vi "Measurement_input_panel.vi"(0 "OK":T4, 2 "setup":T5, 5 "Setup filename":string) -> (11 "Setup filename out":string, 12 "Analysis Info cluster":T8[](array[typedef])=[{"Colour"=0, "Inst type"=enum."Pitot-static tube", "Inst name"="Manometer voltage", "Symbol"="U", "Code name"="", "Extra Info"="U", "Inst Array"=enum."PWA", "Index"=0, "Voltage Index"=0, "Extra Titles"=[], "Extra Values"=[]}, {"Colour"=0, "Inst type"=enum."Pitot-static tube", "Inst name"="Manometer voltage", "Symbol"="U", "Code name"="", "Extra Info"="U", "Inst Array"=enum."PWA", "Index"=0, "Voltage Index"=0, "Extra Titles"=[], "Extra Values"=[]}, {"Colour"=0, "Inst type"=enum."Pitot-static tube", "Inst name"="Manometer voltage", "Symbol"="U", "Code name"="", "Extra Info"="U", "Inst Array"=enum."PWA", "Index"=0, "Voltage Index"=0, "Extra Titles"=[], "Extra Values"=[]}], 19 "Board type":T10=enum."NB-MIO-16H")   [LabVIEW 2010]
uses:
  Controls/Inst_type.ctl
  Controls/Board_Types.ctl
  Controls/Analysis_info_cluster.ctl
  Controls/Instrument_Array.ctl
  Controls/Setup.ctl
  Controls/ok_button.ctl
  Controls/Trigger_Mode.ctl
  Controls/PWA_Data.ctl
  Controls/Post_Process.ctl
  Controls/App_Global.ctl
  Controls/Ch_and_Spans.ctl
  Globals/Meas_global.vi
  Globals/Trav_pos_global.vi
  Globals/Constants_global.vi
  Globals/LDA_meas_global_1.vi
  Globals/Preference_global.vi
panel:
  in  "Select Duplicate Channels":bool
  in  "PWA Data":T1
  out "Inst type":T2
  in  "Edit temp and Press":bool
  out "Abs Press (mbar)":dbl=1013.0 format="%.1f"
  out "Temp (deg C)":dbl=21.0 format="%.1f"
  in  "Trigger mode":T3
  in  "Select Plug Ins":bool
  in  "Sync Delay Time (ms)":dbl=24.0 format="%.2f"
  out "XW Present?":bool
  out "Read Setup File?":bool
  out "Setup File":path
  out "Setup Paths":path[](array[path])
  in  "Select Local ADAM Channels":bool
  out "Local ADAM Channels":string[](array[string])
  in  "stop":bool
  out "Notes":string
  in  "Setup filename selector":u16(ring) items=["Current_Setup.xls", "5168SetupTakeZeroes.xls", "5168FIDRawVoltsSanityCheck.xls", "5168Setup6min.xls", "5168Setup5min.xls", "5168Setup4min.xls", "5168Setup3min.xls", "5168SetupTapped1to1cal.xls", "5168SetupTappedNoPuffs1to1cal.xls", "5168SetupTappedNoPuffs.xls", "5168SetupTapped.xls", "5168Setup2.xls", "5168FIDcheck.xls", "5168Setup1.xls"]
  in  "Synchronise Analogue channels with LDA":bool
  in  "LDA set up":T6={"dimensions"=enum."2D", "Arrival spacing"=FALSE, "Transit time"=FALSE}
  in  "LDA data":enum16{"No LDA data", "Take LDA data"}(ring)=enum."Take LDA data"
  in  "Cross wire":T7(ring)
  in  "Acquisition Method":T10=enum."NB-MIO-16H"
  in  "No of Analogue inst":i32=1
  in  "Ch & spans choices":T11(array[cluster]) {"D" format="%.2f"; "Ch No" min=0; "low limit" min=-10 max=10 format="%.2f"; "high limit" min=-10 max=10 format="%.2f"}
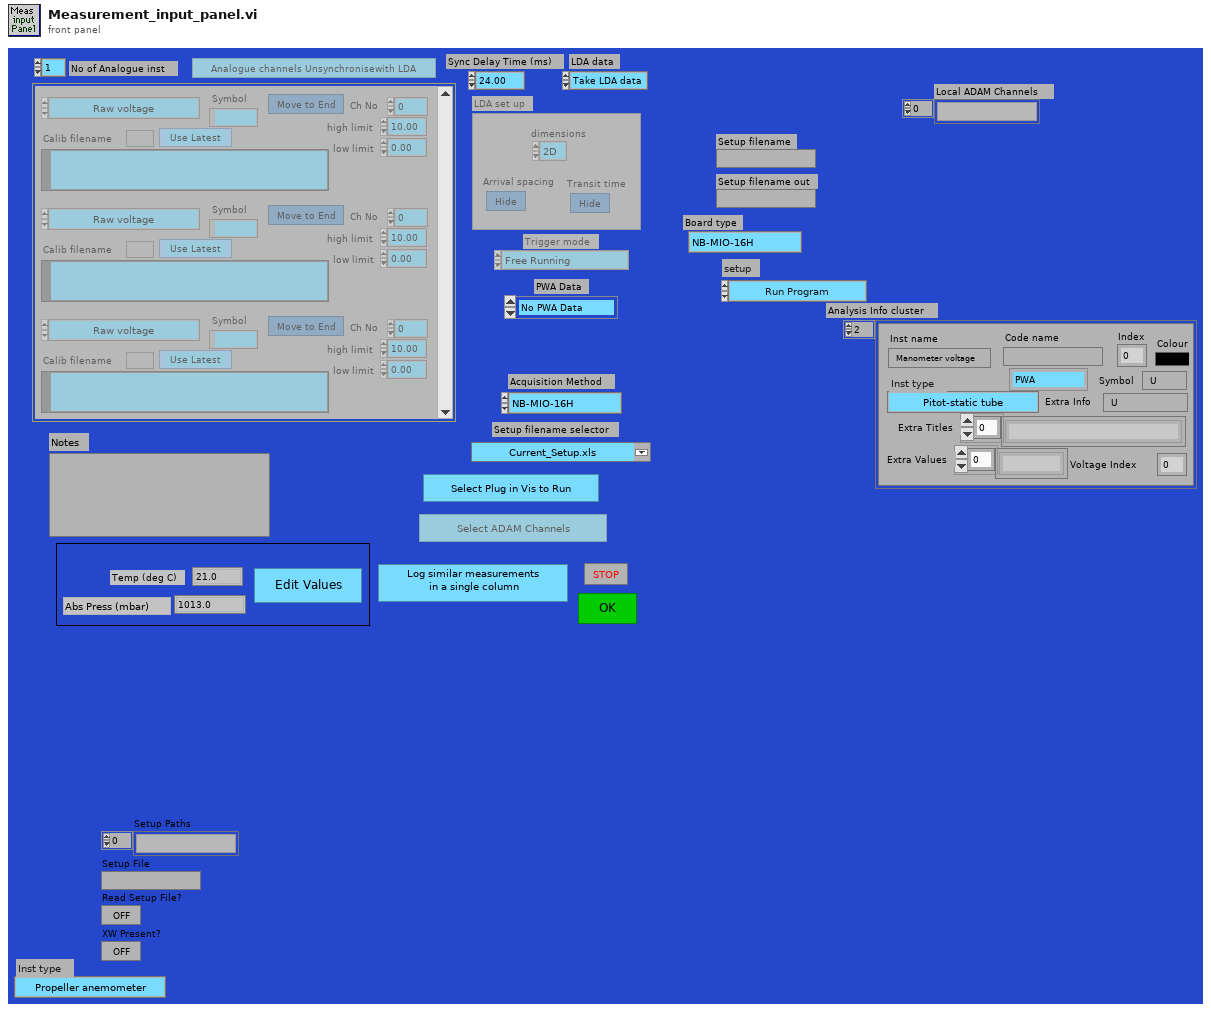
[diagram p1: front panel]
types:
  T1 = typedef "PWA_Data.ctl" = enum16{"No PWA Data", "One Ch PWA"}
  T2 = typedef "Inst_type.ctl" = enum16{"Propeller anemometer", "Raw voltage", "Pressure Transducer", "Pitot-static tube", "Preston tube", "Hot wire", "Cross wire 1", "Cross wire 2", "Generic Linear", "Generic Polynomial", "Generic BackPoly", "Fast FID", "Thermocouple", "Cold wire", "Pulsed Wire", "LDA Vel", "LDA Tran time", "LDA Arr time"}
  T3 = typedef "Trigger_Mode.ctl" = enum16{"Free Running", "Start on Trigger", "Trigger Every Block", "Trigger Every Sample"}
  T4 = typedef "ok_button.ctl" = bool
  T5 = typedef "Setup.ctl" = enum16{"Run Program", "Show Setup", "Save Current Setup", "Setup Front Panel"}
  T6 = cluster{"dimensions":enum16{"1D", "2D"}, "Arrival spacing":bool, "Transit time":bool}
  T7 = enum16{"2nd component as calculated", "2nd component multipled by -1"}
  T8 = typedef "Analysis_info_cluster.ctl" = cluster{"Colour":u32, "Inst type":T2, "Inst name":string, "Symbol":string, "Code name":string, "Extra Info":string, "Inst Array":T9, "Index":i32, "Voltage Index":i32, "Extra Titles":string[], "Extra Values":string[]}
  T9 = typedef "Instrument_Array.ctl" = enum16{"PWA", "LDA", "Analogue"}
  T10 = typedef "Board_Types.ctl" = enum16{"Simulate", "NB-MIO-16H", "PCI-MIO-16E", "6000E Series", "USB-92xx", "ADC488", "Lab-NB", "NB-DIO-24", "NI-DAQmx", "Local ADAM", "Server Channels"}
  T11 = cluster{"high limit":sgl, "low limit":sgl, "Ch No":i16, "Calib filename":path, "Inst type":T2, "Symbol":string, "Move channel":bool, "Use Latest":bool, "D":dbl, "Ch Name":string}[]
  T12 = typedef "Post_Process.ctl" = enum16{"Take New Data", "Post Process Raw Data File"}
  T13 = cluster{"high limit (10V)":sgl, "low limit (-10V)":sgl, "Ch No":i16, "Calib filename":path, "Inst type":T2, "Symbol":string, "Move channel":bool, "Use Latest":bool, "D":dbl, "Ch Name":string}
  T14 = typedef "App_Global.ctl" = enum16{"Read Global", "Write to Global", "Initialise Array"}
  T15 = typedef "Ch_and_Spans.ctl" = cluster{"high limit (10V)":sgl, "low limit (-10V)":sgl, "Ch No":i16, "Var name":string, "Use Latest Calib":bool}
  T16 = enum16{"Zero or one", "One", "Zero or more", "One or more"}
  T17 = typedef "Traverse_cluster.ctl" = cluster{"Start X":dbl, "Start Y":dbl, "Start Z":dbl, "End X":dbl, "End Y":dbl, "End Z":dbl, "No. of pts.":i32, "Spacing":T18, "Filename":path, "Tunnel Speed":dbl, "Averaging time (min)":dbl, "Extra Commands":string, "Specific Arguments":string, "Emission Rate (l/min)":dbl, "Trace Gas Concentration (%)":dbl, "Density Ratio":string, "Comments":string, "Row No":i32, "Row Type Selector":T19, "Completion time":string, "Row Duration (mins)":dbl, "No. of Valid pts.":i32, "Meas Setup File":string}
  T18 = typedef "Spacing.ctl" = enum16{"Linear", "Log", "Gauss", "Specified", "N/A"}
  T19 = typedef "Multi_run_mode.ctl" = enum16{"Move Traverse Only", "Set Tunnel Speed Only", "Set Source Only", "Set Measurement Conditions", "Single Measurement", "Vertical Profile", "Lateral Profile", "Longitudinal Profile", "Explore Volume", "Multi-Axis Profile", "Auto Calibrate", "Meas Fast FID Bkgnd", "Check Beam Power", "Scanning Valve Measurement", "Run VI Named:", "Set ADAM Ch", "Wait (minutes)", "Send Message", "Synchronize With:", "Fall Back to this Row", "Turn Off Row Repeating", "Blank Row"}
  T20 = cluster{"high limit (10V)":sgl, "low limit (-10V)":sgl, "Ch No":i16, "Calib filename":path, "Inst type":T2, "Symbol":string, "Move channel":bool, "Use Latest":bool, "D":dbl, "Ch Name":string}[]
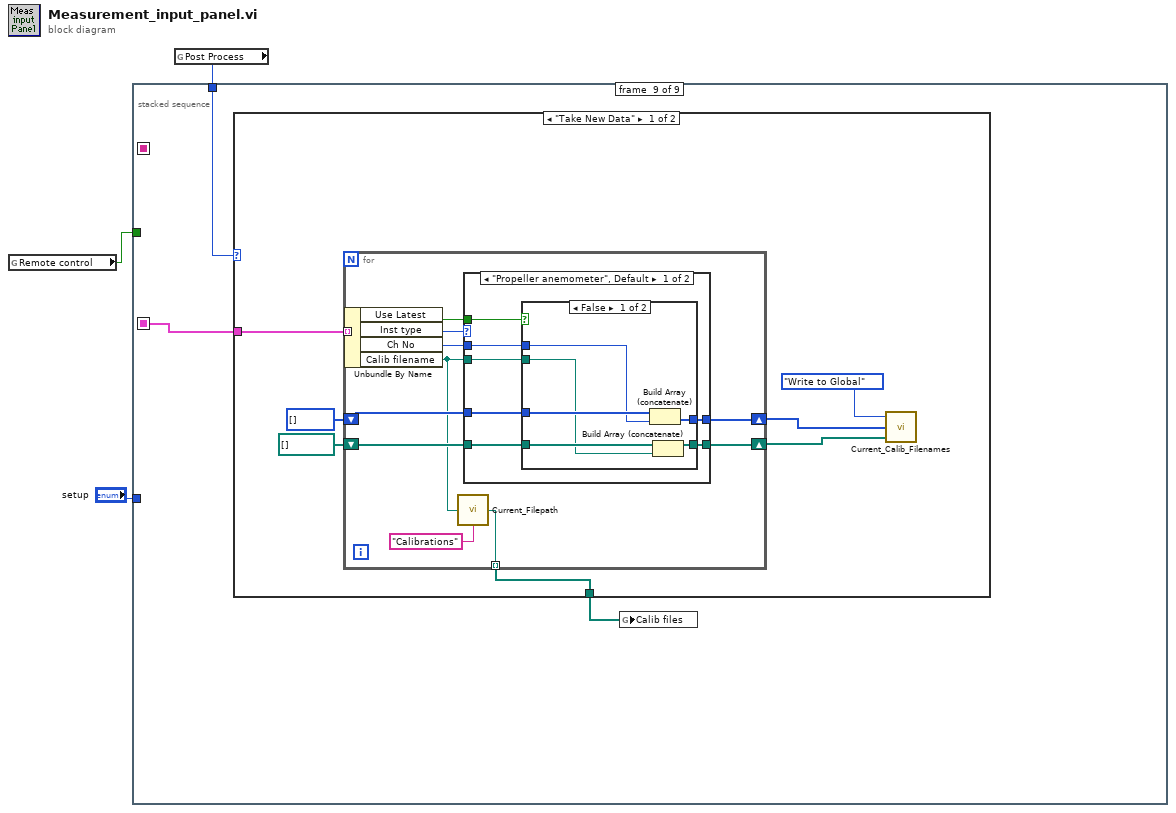
[diagram p0: block diagram]
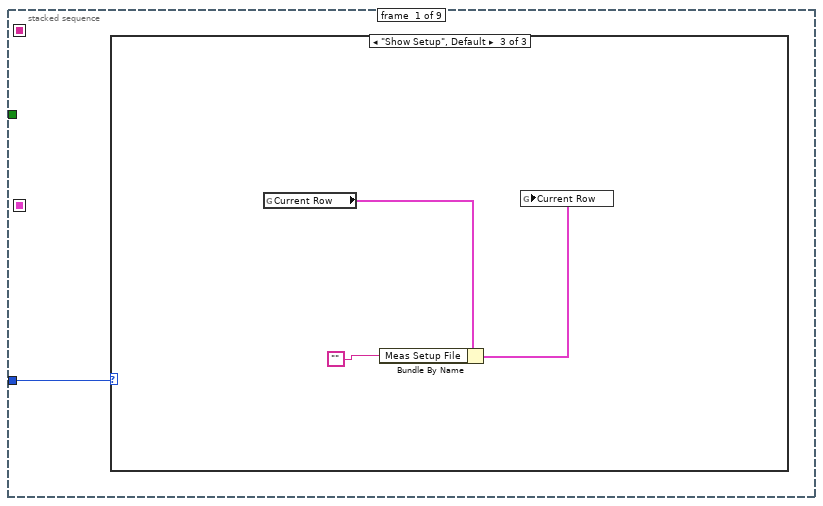
[diagram p2: hidden frame]
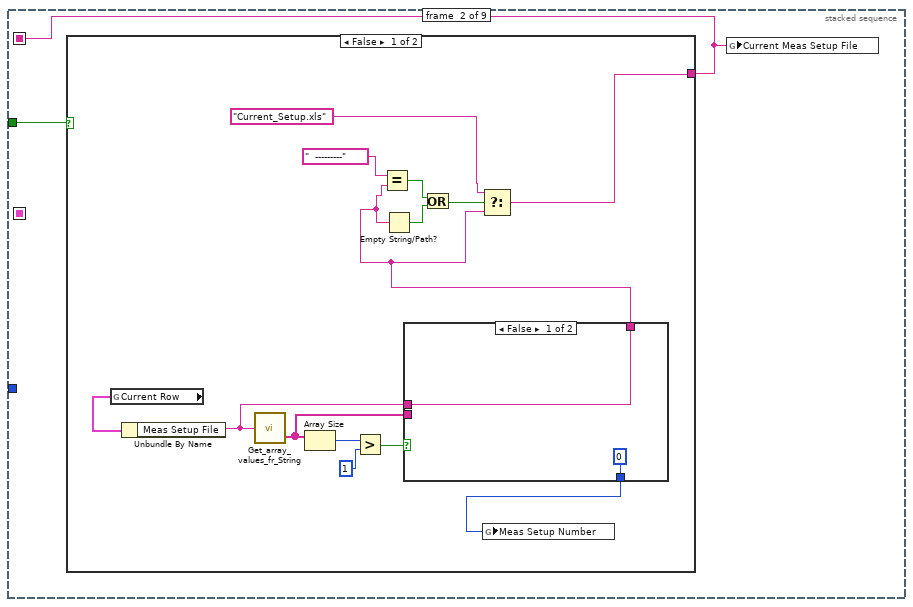
[diagram p5: hidden frame]
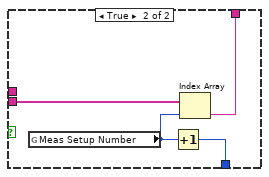
[diagram p6: hidden frame]
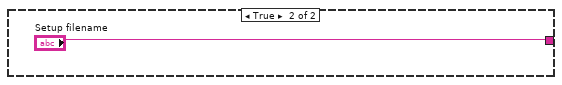
[diagram p7: hidden frame]
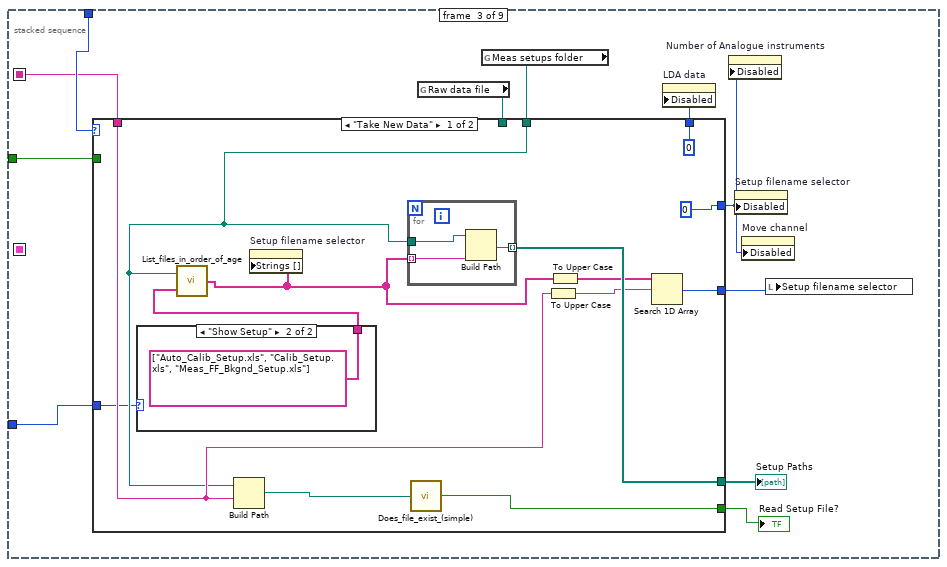
[diagram p8: hidden frame]
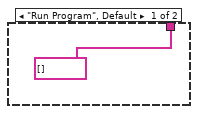
[diagram p9: hidden frame]
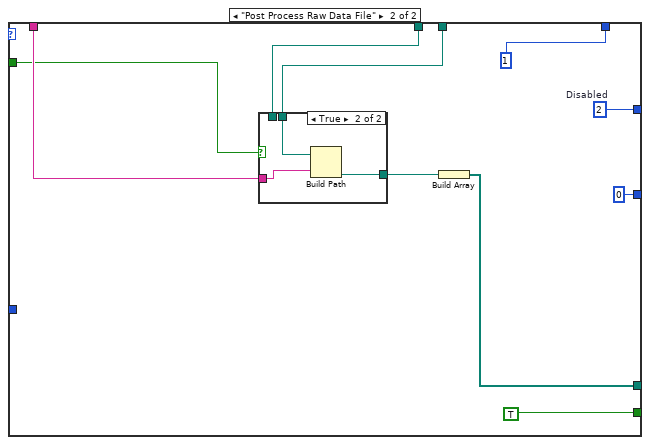
[diagram p10: hidden frame]
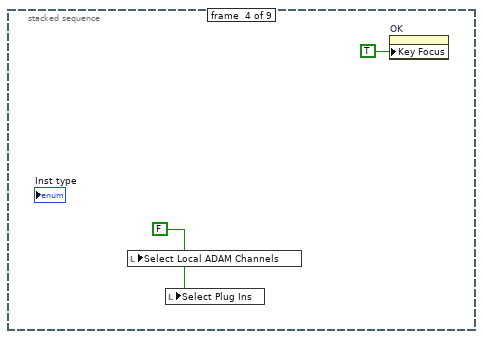
[diagram p12: hidden frame]
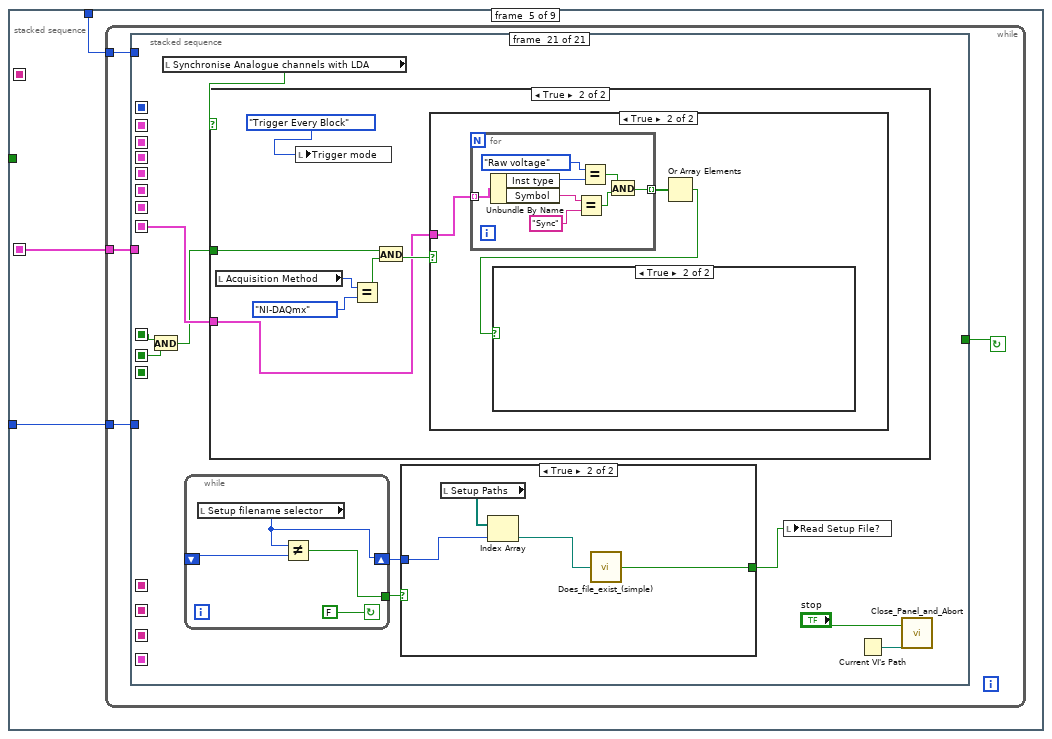
[diagram p13: hidden frame]
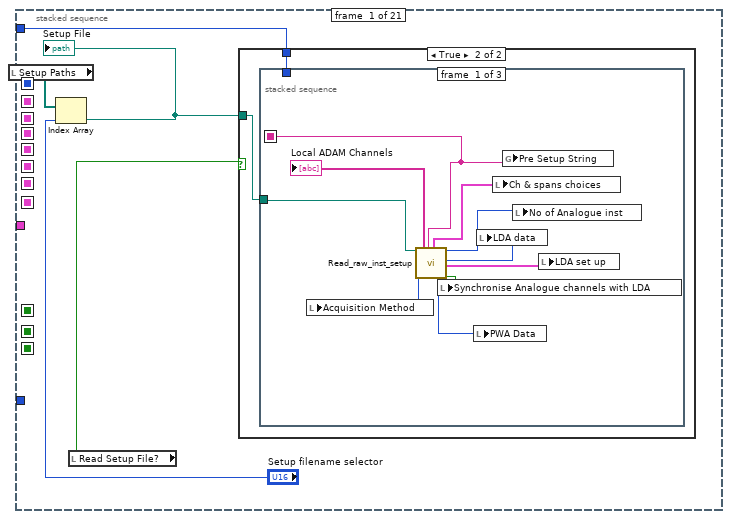
[diagram p14: hidden frame]
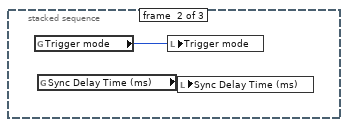
[diagram p16: hidden frame]
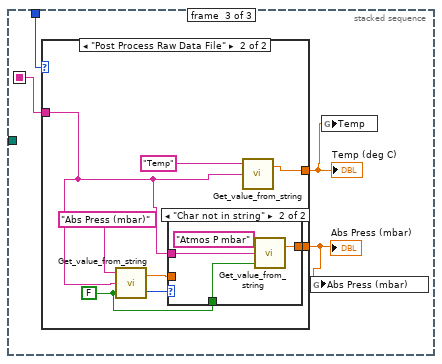
[diagram p17: hidden frame]
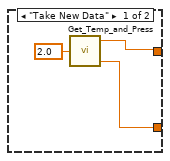
[diagram p18: hidden frame]
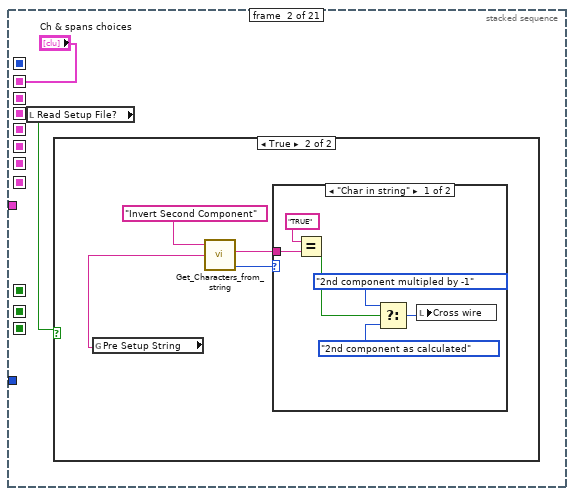
[diagram p20: hidden frame]
diagram:
  n1 = global read "Meas_global.vi" "Remote control"() -> (w1:bool)
  n2 = global read "Meas_global.vi" "Post Process"() -> (w3:T12)
  n3 = stacked-sequence {
    seq-local: [_ _ _ _ w78 _ _ _ _] -> [_ _ _ _ _ _ w762 _ w888]
    seq-local: [_ w8 _ _ _ _ _ _ _] -> [_ _ w31 _ _ _ w761 _ _]
    tunnel: w3 -> [_ _ w41 _ w77 _ _ _ w887]
    tunnel: "setup" -> [w4 _ w33 _ w76 _ w763 _ _]
    tunnel: w1 -> [_ w9 w32 _ _ _ _ _ _]
    frame #0 {
      n4 = case shown="\"Show Setup\", Default" w4 {
        frame "Run Program" {
        }
        frame "Setup Front Panel" {
        }
        frame "Show Setup", Default {
          n5 = global read "Trav_pos_global.vi" "Current Row"() -> (w7:T17)
          n6 = Bundle By Name(cluster=w7, "Meas Setup File"="") -> (w6:T17)
          n7 = global write "Trav_pos_global.vi" "Current Row"(w6) -> ()
        }
      }
    }
    frame #1 {
      n8 = case shown="False" w9 {
        tunnel: [w22 "Setup filename"] -> w8
        frame False {
          n9 = global read "Trav_pos_global.vi" "Current Row"() -> (w18:T17)
          n10 = Unbundle By Name(w18) -> ("Meas Setup File"=w12:string)
          n11 = call "Get_array_values_fr_String.vi"("String Value"=w12) -> ("String array"=w11:string[])  [unwired: 1 out]
          n12 = Array Size(array=w11) -> (size(s)=w16:i32)
          n13 = Greater?(x=w16, y=1) -> (0:w14:bool)
          n14 = case shown="False" w14 {
            tunnel: [w25 w28] -> w13
            tunnel: w12 -> [w25 _]
            tunnel: w11 -> [_ w29]
            tunnel: [0 w26] -> w10
            frame False {
            }
            frame True {
              n15 = global read "Trav_pos_global.vi" "Meas Setup Number"() -> (w27:i32)
              n16 = Increment(x=w27) -> (x+1=w26:i32)
              n17 = Index Array(array=w29, index=w27) -> (element=w28:string)
            }
          }
          n18 = Equal?(x="  ---------" ("f"), y=w13) -> (x = y?=w21:bool)
          n19 = Empty String/Path?(string/path=w13) -> (empty?=w20:bool)
          n20 = Or(x=w21, y=w20) -> (x .or. y?=w17:bool)
          n21 = Select(t="Current_Setup.xls", s=w17, f=w13) -> (s? t:f=w22:string)
          n22 = global write "Trav_pos_global.vi" "Meas Setup Number"(w10) -> ()
        }
        frame True {
        }
      }
      n23 = global write "Trav_pos_global.vi" "Current Meas Setup File"(w8) -> ()
    }
    frame #2 {
      n24 = global read "Meas_global.vi" "Raw data file"() -> (w38:path)
      n25 = global read "Constants_global.vi" "Meas setups folder"() -> (w36:path)
      n26 = case shown="\"Take New Data\"" w41 {
        tunnel: [w52 w65] -> w35
        tunnel: [w46 TRUE ("exists")] -> w34
        tunnel: [u8 0 ("Disabled") w61] -> w37
        tunnel: [u8 0 ("Disabled") u8 1 ("Disabled")] -> w40
        tunnel: w31 -> [w51 w67]
        tunnel: [w53 0 ("index of element")] -> w39
        tunnel: w36 -> [w48 w68]
        tunnel: w38 -> [_ w63]
        tunnel: w33 -> [w42 _]
        tunnel: w32 -> [_ w60]
        frame "Take New Data" {
          n27 = case shown="\"Show Setup\"" w42 {
            tunnel: [string[] [] ("file names") string[] ["Auto_Calib_Setup.xls", "Calib_Setup.xls", "Meas_FF_Bkgnd_Setup.xls"] ("file names")] -> w44
            frame "Run Program", Default {
            }
            frame "Show Setup" {
            }
          }
          n28 = call "List_files_in_order_of_age.vi"("Files to Hide"=w44, "Folder"=w48) -> ("file names"=w43:string[])
          n29 = Build Path(base path=w48, name or relative path=w51) -> (appended path=w47:path)
          n30 = property on="Setup filename selector" class="Ring (strict)"("Strings []"=w43) -> ()  [unwired: 2 in, 2 out]
          n31 = for {
            tunnel: [w57] -> w52 mode=indexing
            tunnel: w48 -> [w58]
            tunnel: w43 -> [w59] mode=indexing
            n32 = Build Path(base path=w58, name or relative path=w59) -> (appended path=w57:path)
          }
          n33 = call "Does_file_exist_(simple).vi"("Pathname"=w47) -> ("exists?"=w46:bool)
          n34 = To Upper Case(1:w51) -> (0:w49:string)
          n35 = To Upper Case(1:w43) -> (0:w50:string[])
          n36 = Search 1D Array(1D array=w50, element=w49) -> (index of element=w53:i32)  [unwired: 1 out]
        }
        frame "Post Process Raw Data File" {
          w61 = u8 2  # Disabled
          n37 = case shown="True" w60 {
            tunnel: w68 -> [_ w73]
            tunnel: w67 -> [_ w72]
            tunnel: [w70 w71] -> w66
            tunnel: w63 -> [w70 _]
            frame False {
            }
            frame True {
              n38 = Build Path(base path=w73, name or relative path=w72) -> (appended path=w71:path)
            }
          }
          n39 = Build Array(w66) -> (w65:path[])
        }
      }
      "Setup Paths" <- w35
      "Read Setup File?" <- w34
      n40 = property on="LDA data" class="Enum (strict)"("Disabled"=w40) -> ()  [unwired: 2 in, 2 out]
      n41 = property on="Number of Analogue instruments" class="DigNum (strict)"("Disabled"=w37) -> ()  [unwired: 2 in, 2 out]
      n42 = property on="Setup filename selector" class="Ring (strict)"("Disabled"=w37) -> ()  [unwired: 2 in, 2 out]
      n43 = property on="Move channel" class="Bool (strict)"("Disabled"=w37) -> ()  [unwired: 2 in, 2 out]
      n44 = local write "Setup filename selector"(w39) -> ()
    }
    frame #3 {
      w75 = FALSE ("Select Local ADAM Channels")
      n45 = local write "Select Local ADAM Channels"(w75) -> ()
      n46 = local write "Select Plug Ins"(w75) -> ()
      n47 = property on="OK" class="Bool"("Key Focus"=TRUE) -> ()  [unwired: 2 in, 2 out]
    }
    frame #4 {
      n48 = while {
        tunnel: w76 -> [w79]
        tunnel: w77 -> [w80]
        tunnel: [w82] -> w78
        stop <- w81 continue-if-true
        n49 = stacked-sequence {
          seq-local: [_ _ _ _ _ _ _ _ w270 _ _ _ _ _ _ _ _ _ _ _ _] -> [_ _ _ _ _ _ _ _ _ w337 _ _ _ _ _ _ _ _ _ _ _]
          seq-local: [_ _ _ w159 _ _ _ _ _ _ _ _ _ _ _ _ _ _ _ _ _] -> [_ _ _ _ _ w212 w247 w266 w271 _ _ _ _ _ _ _ _ _ _ _ _]
          seq-local: [_ _ _ _ _ w217 _ _ _ _ _ _ _ _ _ _ _ _ _ _ _] -> [_ _ _ _ _ _ _ _ w272 _ _ _ _ _ _ _ _ _ _ _ _]
          seq-local: [_ _ _ _ _ _ _ _ _ w336 _ _ _ _ _ _ _ _ _ _ _] -> [_ _ _ _ _ _ _ _ _ _ w370 w418 w461 _ _ _ _ _ _ _ _]
          seq-local: [_ _ _ _ _ _ _ _ _ _ w368 _ _ _ _ _ _ _ _ _ _] -> [_ _ _ _ _ _ _ _ _ _ _ w413 _ _ _ _ _ _ _ _ w721]
          seq-local: [_ _ _ _ _ _ _ _ _ _ _ _ _ w490 _ _ _ _ _ _ _] -> [_ _ _ _ _ _ _ _ _ _ _ _ _ _ w509 _ _ _ _ _ _]
          seq-local: [_ _ _ _ _ _ _ _ _ _ _ _ _ _ w505 _ _ _ _ _ _] -> [_ _ _ _ _ _ _ _ _ _ _ _ _ _ _ w531 w537 w600 _ w697 w722]
          seq-local: [_ _ _ _ _ _ _ _ _ _ _ w417 _ _ _ _ _ _ _ _ _] -> [_ _ _ _ _ _ _ _ _ _ _ _ _ w487 _ _ _ _ _ _ _]
          seq-local: [_ _ _ _ _ _ _ _ _ _ _ _ w460 _ _ _ _ _ _ _ _] -> [_ _ _ _ _ _ _ _ _ _ _ _ _ w486 _ _ _ _ _ _ _]
          seq-local: [_ _ _ _ _ _ _ _ _ w330 _ _ _ _ _ _ _ _ _ _ _] -> [_ _ _ _ _ _ _ _ _ _ w367 w414 _ _ _ _ _ _ _ _ w720]
          seq-local: [_ _ _ _ _ _ _ _ _ _ _ _ _ _ _ _ w536 _ _ _ _] -> [_ _ _ _ _ _ _ _ _ _ _ _ _ _ _ _ _ w603 _ _ _]
          seq-local: [_ _ _ _ _ _ _ _ _ _ _ _ _ _ _ _ w535 _ _ _ _] -> [_ _ _ _ _ _ _ _ _ _ _ _ _ _ _ _ _ w602 _ _ _]
          seq-local: [_ _ _ _ _ _ _ _ _ _ _ _ _ _ _ _ w534 _ _ _ _] -> [_ _ _ _ _ _ _ _ _ _ _ _ _ _ _ _ _ w601 _ _ _]
          seq-local: [_ _ _ _ _ _ _ _ _ _ _ _ _ _ _ _ _ w599 _ _ _] -> [_ _ _ _ _ _ _ _ _ _ _ _ _ _ _ _ _ _ w641 _ _]
          seq-local: [_ "Ch & spans choices" _ _ _ _ _ _ _ _ _ _ _ _ _ _ _ _ _ _ _] -> [_ _ _ w142 _ _ _ _ _ _ _ _ _ _ _ w530 _ _ _ _ _]
          tunnel: [_ _ _ _ _ _ _ _ _ _ _ _ _ _ w505 _ _ _ _ _ _] -> w82
          tunnel: [_ _ _ _ _ _ _ _ _ _ _ w415 _ _ _ _ _ _ _ _ _] -> w81
          tunnel: w80 -> [w83 _ w134 w154 _ _ _ _ _ w331 _ w412 _ w489 _ _ _ _ _ w698 _]
          tunnel: w79 -> [_ _ _ _ w198 _ _ _ _ _ _ _ _ w488 _ _ _ _ w643 _ _]
          frame #0 {
            n50 = local read "Setup Paths"() -> (w86:path[])
            n51 = Index Array(array=w86, index="Setup filename selector") -> (element=w87:path)
            "Setup File" <- w87
            n52 = local read "Read Setup File?"() -> (w85:bool)
            n53 = case shown="True" w85 {
              tunnel: w87 -> [_ w89]
              tunnel: w83 -> [_ w88]
              frame False {
              }
              frame True {
                n54 = stacked-sequence {
                  seq-local: [w92 _ _] -> [_ _ w104]
                  tunnel: w89 -> [w95 _ _]
                  tunnel: w88 -> [_ _ w105]
                  frame #0 {
                    n55 = call "Read_raw_inst_setup.vi"("Setup file"=w95) -> ("Board type"=w97:T10, "Local ADAM Channels"=→"Local ADAM Channels":string[], "Setup string"=w92:string, "Ch & spans choices"=w91:T20, "PWA Data"=w90:T1, "Number of Analogue instruments"=w99:i32, "LDA data"=w98:enum16{"No LDA data", "Take LDA data"}, "LDA set up"=w94:T6, "Synchronise Analogue channels with LDA"=w96:bool)  [unwired: 10 out]
                    n56 = local write "Acquisition Method"(w97) -> ()
                    n57 = local write "Synchronise Analogue channels with LDA"(w96) -> ()
                    n58 = local write "PWA Data"(w90) -> ()
                    n59 = local write "LDA data"(w98) -> ()
                    n60 = local write "Ch & spans choices"(w91) -> ()
                    n61 = global write "Meas_global.vi" "Pre Setup String"(w92) -> ()
                    n62 = local write "No of Analogue inst"(w99) -> ()
                    n63 = local write "LDA set up"(w94) -> ()
                  }
                  frame #1 {
                    n64 = global read "Meas_global.vi" "Trigger mode"() -> (w100:T3)
                    n65 = global read "LDA_meas_global_1.vi" "Sync Delay Time (ms)"() -> (w101:dbl)
                    n66 = local write "Trigger mode"(w100) -> ()
                    n67 = local write "Sync Delay Time (ms)"(w101) -> ()
                  }
                  frame #2 {
                    n68 = case shown="\"Post Process Raw Data File\"" w105 {
                      tunnel: w104 -> [_ w111]
                      tunnel: [w106 w110] -> w102
                      tunnel: [w107 w109] -> w103
                      frame "Take New Data" {
                        n69 = call "Get_Temp_and_Press.vi"("Averaging time (mins)"=2.0) -> ("Abs Press (mbar)"=w106:dbl, "Temperature"=w107:dbl)  [unwired: 3 out]
                      }
                      frame "Post Process Raw Data File" {
                        w113 = FALSE ("Show Dialog?")
                        n70 = call "Get_value_from_string.vi"("Show Dialog?"=w113, "Input string"=w111, "Variable name"="Abs Press (mbar)") -> ("Status"=w115:enum16{"Char in string", "Char not in string"}, "Value"=w114:dbl)
                        n71 = case shown="\"Char not in string\"" w115 {
                          tunnel: [w117 w120] -> w110
                          tunnel: w114 -> [w117 _]
                          tunnel: w113 -> [_ w119]
                          tunnel: w111 -> [_ w118]
                          frame "Char in string" {
                          }
                          frame "Char not in string" {
                            n72 = call "Get_value_from_string.vi"("Show Dialog?"=w119, "Input string"=w118, "Variable name"="Atmos P mbar") -> ("Value"=w120:dbl)  [unwired: 1 out]
                          }
                        }
                        n73 = call "Get_value_from_string.vi"("Input string"=w111, "Variable name"="Temp") -> ("Value"=w109:dbl)  [unwired: 1 in, 1 out]
                      }
                    }
                    "Abs Press (mbar)" <- w102
                    "Temp (deg C)" <- w103
                    n74 = global write "Meas_global.vi" "Abs Press (mbar)"(w102) -> ()
                    n75 = global write "Meas_global.vi" "Temp"(w103) -> ()
                  }
                }
              }
            }
          }
          frame #1 {
            n76 = local read "Read Setup File?"() -> (w123:bool)
            n77 = case shown="True" w123 {
              frame False {
              }
              frame True {
                n78 = global read "Meas_global.vi" "Pre Setup String"() -> (w126:string)
                n79 = call "Get_Characters_from_string.vi"("Input string"=w126, "Variable name"="Invert Second Component") -> ("Status"=w125:enum16{"Char in string", "Char not in string"}, "Value"=w124:string)  [unwired: 1 in]
                n80 = case shown="\"Char in string\"" w125 {
                  tunnel: w124 -> [w133 _]
                  frame "Char in string" {
                    n81 = Equal?(x="TRUE", y=w133) -> (x = y?=w129:bool)
                    n82 = Select(t=T7."2nd component multipled by -1" ("Cross wire/LDA"), s=w129, f=T7."2nd component as calculated" ("Cross wire/LDA")) -> (s? t:f=w131:T7)
                    n83 = local write "Cross wire"(w131) -> ()
                  }
                  frame "Char not in string" {
                  }
                }
              }
            }
          }
          frame #2 {
            n84 = case shown="True" "Edit temp and Press" {
              tunnel: w134 -> [_ w136]
              frame False {
              }
              frame True {
                n85 = case shown="\"Take New Data\"" w136 {
                  frame "Take New Data" {
                    n86 = stacked-sequence {
                      frame #0 {
                        w137 = TRUE  # Wait until done
                        n87 = call "Run_Enter_Temp.vi"("Wait until done"=w137) -> ()  [unwired: 1 out]
                      }
                      frame #1 {
                        n88 = call "Get_Temp_and_Press.vi"("Averaging time (mins)"=2.0) -> ("Abs Press (mbar)"=w138:dbl, "Temperature"=w139:dbl)  [unwired: 3 out]
                        n89 = local write "Temp (deg C)"(w139) -> ()
                        n90 = local write "Abs Press (mbar)"(w138) -> ()
                      }
                    }
                  }
                  frame "Post Process Raw Data File" {
                  }
                }
              }
            }
          }
          frame #3 {
            w150 = u8 0  # Disabled
            n91 = local read "Read Setup File?"() -> (w141:bool)
            n92 = Equal?(x=w154, y=Post_Process."Take New Data" ("Post Process")) -> (x = y?=w153:bool)
            n93 = local read "Acquisition Method"() -> (w147:T10)
            n94 = Equal?(x=w147, y=Board_Types."Local ADAM" ("Board type")) -> (x = y?=w144:bool)
            n95 = Equal?(x=Board_Types."Server Channels" ("Board type"), y=w147) -> (x = y?=w145:bool)
            n96 = Or(x=w144, y=w145) -> (x .or. y?=w143:bool)
            n97 = And(x=w141, y=w143) -> (x .and. y?=w158:bool)
            n98 = Or(x="Select Local ADAM Channels", y=w158) -> (x .or. y?=w151:bool)
            n99 = And(x=w153, y=w151) -> (x .and. y?=w152:bool)
            n100 = case shown="True" w152 {
              tunnel: [w161 w164] -> w159
              tunnel: w142 -> [w161 w165]
              tunnel: "Select Local ADAM Channels" -> [_ w163]
              tunnel: w144 -> [_ w162]
              frame False {
              }
              frame True {
                n101 = local read "Local ADAM Channels"() -> (w167:string[])
                n102 = stacked-sequence {
                  seq-local: [_ w176 _ _ _] -> [_ _ w182 w195 _]
                  seq-local: [_ w180 _ _ _] -> [_ _ w186 _ _]
                  seq-local: [T13 {"high limit (10V)"=10.0, "low limit (-10V)"=0.0, "Ch No"=0, "Calib filename"=path "", "Inst type"=enum."Raw voltage", "Symbol"="", "Move channel"=FALSE, "Use Latest"=FALSE, "D"=0.0, "Ch Name"=""} _ _ _ _] -> [_ w172 _ _ _]
                  seq-local: [_ w169 _ _ _] -> [_ _ w184 _ _]
                  tunnel: w167 -> [_ w179 _ _ _]
                  tunnel: [_ w180 _ _ _] -> w166
                  tunnel: w165 -> [_ w171 _ _ _]
                  tunnel: [_ _ w185 _ _] -> w164
                  tunnel: w163 -> [_ w181 _ _ w196]
                  tunnel: w162 -> [_ w177 w183 _ _]
                  frame #0 {
                  }
                  frame #1 {
                    n103 = Array Size(array=w171) -> (size(s)=w174:i32)
                    n104 = Array Subset(array=w179, length=w174) -> (w178:string[])  [unwired: 1 in]
                    n105 = call "Get_local_ADAM_Chs.vi"("Local ADAM?"=w177, "Show setup"=w181, "Desired Local ADAM Channels"=w178) -> ("Choosen Channels"=w180:string[], "Ch Indicies Choosen"=w176:i32[])
                    n106 = Array Size(array=w176) -> (size(s)=w175:i32)
                    n107 = Subtract(x=w175, y=w174) -> (x-y=w173:i32)
                    n108 = Initialize Array(w172, w173) -> (w170:T20)
                    n109 = Build Array (concatenate)(w171, w170) -> (w169:T20)
                  }
                  frame #2 {
                    n110 = for {
                      tunnel: [w193] -> w185 mode=indexing
                      tunnel: w186 -> [w192] mode=indexing
                      tunnel: w184 -> [w191] mode=indexing
                      tunnel: w183 -> [w190]
                      tunnel: w182 -> [w189] mode=indexing
                      i -> [w188]
                      n111 = Select(t=w189, s=w190, f=w188) -> (s? t:f=w187:i32)
                      n112 = Bundle By Name(cluster=w191, "Ch No"=w187, "Ch Name"=w192) -> (w193:T13)
                    }
                  }
                  frame #3 {
                    n113 = Array Size(array=w195) -> (size(s)=w194:i32)
                    n114 = local write "No of Analogue inst"(w194) -> ()
                  }
                  frame #4 {
                    n115 = case shown="True" w196 {
                      frame False {
                      }
                      frame True {
                        n116 = local write "Select Local ADAM Channels"(FALSE ("Select Local ADAM Channels")) -> ()
                      }
                    }
                  }
                }
                n117 = local write "Local ADAM Channels"(w166) -> ()
              }
            }
            n118 = Select(t=w150, s=w143, f=u8 2 ("Disabled")) -> (s? t:f=w148:u8)
            n119 = property on="Ch Name" class="Str"("Visible"=w143) -> ()  [unwired: 2 in, 2 out]
            n120 = property on="Select Local ADAM Channels" class="Bool (strict)"("Disabled"=w148) -> ()  [unwired: 2 in, 2 out]
            n121 = Not(x=w143) -> (.not. x?=w156:bool)
            n122 = property on="high limit" class="DigNum (strict)"("Visible"=w156) -> ()  [unwired: 2 in, 2 out]
            n123 = property on="low limit" class="DigNum (strict)"("Visible"=w156) -> ()  [unwired: 2 in, 2 out]
          }
          frame #4 {
            n124 = case shown="True" "Select Plug Ins" {
              tunnel: w198 -> [_ w200]
              frame False {
              }
              frame True {
                n125 = stacked-sequence {
                  tunnel: w200 -> [w201 _]
                  frame #0 {
                    w205 = TRUE  # Show Panel?
                    n126 = global read "Meas_global.vi" "Pre Setup String"() -> (w204:string)
                    n127 = local write "Select Plug Ins"(FALSE ("Select Local ADAM Channels")) -> ()
                    n128 = call "Choose_Plug_In_to_Run.vi"("setup"=w201, "Show Panel?"=w205, "Setup String In"=w204) -> ("Setup String Out"=w203:string)  [unwired: 1 out]
                    n129 = global write "Meas_global.vi" "Pre Setup String"(w203) -> ()
                  }
                  frame #1 {
                    n130 = Current VI's Path() -> (path=w207:path)
                    n131 = call "Open_Close_Front_Panel.ph.vi"("Front Panel Window:Open"=TRUE, "VI path"=w207) -> ()  [unwired: 2 out]
                  }
                }
              }
            }
          }
          frame #5 {
            n132 = Initialize Array(0) -> (w219:i32[])  [unwired: 1 out]
            n133 = for {
              shift-right: [w226] -> w215
              shift-left: w219 -> [w227]
              tunnel: [w225] -> w213 mode=indexing
              tunnel: w212 -> [w224] mode=indexing
              tunnel: [w222] -> w211 mode=indexing
              n134 = Unbundle By Name(w224) -> ("Inst type"=w221:T2)
              n135 = case shown="\"Cross wire 1\"" w221 {
                tunnel: w227 -> [w231 w235 w237 w241]
                tunnel: [w230 w234 w237 w240] -> w226
                tunnel: [FALSE TRUE FALSE FALSE] -> w225
                frame "Propeller anemometer", Default {
                  n136 = Build Array (concatenate)(w231, 1) -> (w230:i32[])
                }
                frame "Cross wire 1" {
                  n137 = Build Array (concatenate)(w235, 2) -> (w234:i32[])
                }
                frame "Cross wire 2" {
                }
                frame "LDA Vel" {
                  n138 = Build Array (concatenate)(w241, 1) -> (w240:i32[])
                }
              }
              n139 = Equal?(x=w221, y=Inst_type."Preston tube" ("Inst type")) -> (x = y?=w222:bool)
            }
            n140 = Build Array (concatenate)(w215, 1) -> (w214:i32[])
            n141 = Array Subset(array=w214, length="No of Analogue inst") -> (w218:i32[])  [unwired: 1 in]
            n142 = Add Array Elements(numeric array=w218) -> (sum=w217:i32)
            n143 = Or Array Elements(Boolean array=w213) -> (logical OR=→"XW Present?":bool)
            n144 = Or Array Elements(Boolean array=w211) -> (logical OR=w209:bool)
            n145 = property on="D" class="DigNum (strict)"("Visible"=w209) -> ()  [unwired: 2 in, 2 out]
          }
          frame #6 {
            n146 = local read "Acquisition Method"() -> (w245:T10)
            n147 = Equal?(x=w245, y=Board_Types."NB-MIO-16H" ("Board type")) -> (x = y?=w243:bool)
            n148 = for {
              tunnel: w247 -> [w252] mode=indexing
              shift-right: [w250] -> w242
              shift-left: "" -> [w249]
              tunnel: w243 -> [w248]
              n149 = Unbundle By Name(w252) -> ("Inst type"=w251:T2)
              n150 = case shown="\"Cross wire 1\"" w251 {
                tunnel: [w254 w261] -> w250
                tunnel: w249 -> [w255 w261]
                tunnel: w248 -> [w253 _]
                frame "Cross wire 1" {
                  n151 = case shown="True" w253 {
                    tunnel: w255 -> [w256 w260]
                    tunnel: [w256 w259] -> w254
                    frame False {
                    }
                    frame True {
                      n152 = Concatenate Strings(w260, "WARNING!\nCheck that sample and hold is working for the cross wire channels. It will affect your results!\n", "\r") -> (w259:string)
                    }
                  }
                }
                frame "Generic Linear", Default {
                }
              }
            }
            "Notes" <- w242
          }
          frame #7 {
            n153 = local read "Acquisition Method"() -> (→"Board type":T10)
            n154 = Array Size(array=w266) -> (size(s)=w265:i32)
            n155 = Not Equal To 0?(x=w265) -> (x != 0?=w264:bool)
            n156 = case shown="True" w264 {
              tunnel: [enum16{"No Analogue data", "Take Analogue data"}."No Analogue data" ("Analogue data") enum16{"No Analogue data", "Take Analogue data"}."Take Analogue data" ("Analogue data")] -> w263
              frame False {
              }
              frame True {
              }
            }
            n157 = global write "Meas_global.vi" "Analogue data"(w263) -> ()
          }
          frame #8 {
            n158 = Index Array(array=w271, index=0) -> (element=w276:T13)
            n159 = Initialize Array(w276) -> (w274:T20)  [unwired: 1 out]
            n160 = Build Array (concatenate)(w271, w276) -> (w275:T20)
            n161 = for {
              N: w272 -> [_]
              tunnel: w275 -> [w284] mode=indexing
              shift-right: [w285] -> w270
              shift-left: w274 -> [w279]
              tunnel: Inst_type."Cross wire 2" ("Inst type") -> [w277]
              shift-right: [w283] -> _
              shift-left: _ -> [w282]
              tunnel: w275 -> [w281]
              n162 = Unbundle By Name(w284) -> ("Inst type"=w283:T2)
              n163 = Array Size(array=w279) -> (size(s)=w278:i32)
              n164 = Increment(x=w278) -> (x+1=w280:i32)
              n165 = case shown="\"Cross wire 1\"" w283 {
                tunnel: [w294 w315 w327] -> w285
                tunnel: w279 -> [w295 w317 w329]
                tunnel: w284 -> [w291 w318 w328]
                tunnel: w277 -> [w293 w322 _]
                tunnel: w282 -> [_ w321 _]
                tunnel: w281 -> [w298 _ _]
                tunnel: w280 -> [w297 _ _]
                frame "Cross wire 1" {
                  n166 = Index Array(array=w298, index=w297) -> (element=w292:T13)
                  n167 = Unbundle By Name(w292) -> ("Inst type"=w296:T2, "high limit (10V)"=w289:sgl, "low limit (-10V)"=w288:sgl, "Ch No"=w287:i16, "Symbol"=w286:string)
                  n168 = Unbundle By Name(w291) -> ("Calib filename"=w290:path)
                  n169 = case shown="\"Generic Linear\", Default" w296 {
                    tunnel: w295 -> [w308 w314]
                    tunnel: [w307 w313] -> w294
                    tunnel: w293 -> [w300 w309]
                    tunnel: w290 -> [w306 w312]
                    tunnel: w291 -> [w304 w310]
                    tunnel: w292 -> [_ _]
                    tunnel: w289 -> [w303 _]
                    tunnel: w288 -> [w302 _]
                    tunnel: w287 -> [w301 _]
                    tunnel: w286 -> [w299 _]
                    frame "Cross wire 2" {
                      n170 = Bundle By Name(cluster=w304, "Calib filename"=w306, "Inst type"=w300, "high limit (10V)"=w303, "low limit (-10V)"=w302, "Ch No"=w301, "Symbol"=w299) -> (w305:T13)
                      n171 = Build Array (concatenate)(w308, w304, w305) -> (w307:T20)
                    }
                    frame "Generic Linear", Default {
                      n172 = Bundle By Name(cluster=w310, "Calib filename"=w312, "Inst type"=w309) -> (w311:T13)
                      n173 = Build Array (concatenate)(w314, w310, w311) -> (w313:T20)
                    }
                  }
                }
                frame "Cross wire 2" {
                  n174 = Decrement(x=w322) -> (x-1=w320:T2)
                  n175 = Equal?(x=w320, y=w321) -> (x = y?=w319:bool)
                  n176 = Bundle By Name(cluster=w318, "Inst type"=w320) -> (w316:T13)
                  n177 = case shown="False" w319 {
                    tunnel: w318 -> [_ _]
                    tunnel: w317 -> [w325 w326]
                    tunnel: w316 -> [w324 _]
                    tunnel: [w323 w326] -> w315
                    frame False {
                      n178 = Build Array (concatenate)(w325, w324) -> (w323:T20)
                    }
                    frame True {
                    }
                  }
                }
                frame "Generic Linear", Default {
                  n179 = Build Array (concatenate)(w329, w328) -> (w327:T20)
                }
              }
            }
          }
          frame #9 {
            # "Order the channel properly for the Lab-NB"
            n180 = case shown="\"NI-DAQmx\"" "Acquisition Method" {
              tunnel: [w339 w341 w343 w345 w347 w349 w351 w354 w362 w363 w365] -> w336
              tunnel: w337 -> [w339 w341 w343 w345 w347 w349 w351 w353 w362 w363 w365]
              tunnel: [w338 w340 w342 w344 w346 w348 w350 w352 w361 w364 w366] -> w334
              tunnel: [w338 w340 w342 w344 w346 w348 w350 w352 w361 w364 w366] -> w333
              frame "Simulate" {
                w338 = TRUE
              }
              frame "NB-MIO-16H" {
                w340 = TRUE
              }
              frame "PCI-MIO-16E" {
                w342 = TRUE
              }
              frame "6000E Series" {
                w344 = TRUE
              }
              frame "USB-92xx" {
                w346 = TRUE
              }
              frame "NI-DAQmx" {
                w348 = TRUE
              }
              frame "ADC488" {
                w350 = TRUE
              }
              frame "Lab-NB" {
                w352 = TRUE
                n181 = for {
                  N -> [w358]
                  tunnel: w353 -> [w355] mode=indexing
                  tunnel: [w356] -> w354 mode=indexing
                  i -> [w360]
                  n182 = Increment(x=w360) -> (x+1=w359:i32)
                  n183 = Subtract(x=w358, y=w359) -> (x-y=w357:i32)
                  n184 = Bundle By Name(cluster=w355, "Ch No"=w357) -> (w356:T13)
                }
              }
              frame "NB-DIO-24" {
                w361 = FALSE
              }
              frame "Local ADAM" {
                w364 = FALSE
              }
              frame "Server Channels" {
                w366 = FALSE
              }
            }
            n185 = Equal?(x=w331, y=Post_Process."Take New Data" ("Post Process")) -> (x = y?=w330:bool)
            n186 = property on="high limit" class="DigNum (strict)"("Visible"=w334) -> ()  [unwired: 2 in, 2 out]
            n187 = property on="low limit" class="DigNum (strict)"("Visible"=w333) -> ()  [unwired: 2 in, 2 out]
          }
          frame #10 {
            n188 = case shown="True" "OK" {
              tunnel: w370 -> [_ w384]
              tunnel: [FALSE w383] -> w368
              tunnel: w367 -> [_ w372]
              frame False {
              }
              frame True {
                n189 = for {
                  tunnel: w384 -> [w396] mode=indexing
                  tunnel: [w394] -> w378 mode=indexing
                  tunnel: [w390] -> w382 mode=indexing
                  n190 = Unbundle By Name(w396) -> ("high limit (10V)"=w399:sgl, "low limit (-10V)"=w398:sgl, "Ch No"=w395:i16, "Inst type"=w393:T2, "Symbol"=w392:string)
                  n191 = Number To Decimal String(number=w393) -> (decimal integer string=w391:string)  [unwired: 1 out]
                  n192 = Concatenate Strings(w391, w392) -> (w390:string)
                  n193 = Greater Or Equal?(x=w399, y=w398) -> (x >= y?=w397:bool)
                  n194 = case shown="\"Propeller anemometer\", Default" w393 {
                    tunnel: w397 -> [w402 _ _ _]
                    tunnel: w395 -> [w401 _ _ _]
                    tunnel: [w400 TRUE TRUE TRUE] -> w394
                    frame "Propeller anemometer", Default {
                      n195 = case shown="True" w402 {
                        tunnel: w401 -> [w405 _]
                        tunnel: [FALSE TRUE] -> w400
                        frame False {
                          n196 = Number To Decimal String(number=w405) -> (decimal integer string=w404:string)  [unwired: 1 out]
                          n197 = Concatenate Strings("Error in input limits for Channel No ", w404) -> (w406:string)
                          n198 = One Button Dialog(message=w406) -> ()  [unwired: 2 out]
                        }
                        frame True {
                        }
                      }
                    }
                    frame "LDA Vel" {
                    }
                    frame "LDA Tran time" {
                    }
                    frame "LDA Arr time" {
                    }
                  }
                }
                n199 = call "Analyse_string_array.vi"("String array"=w382) -> ("Frequency"=w381:i32[])  [unwired: 2 out]
                n200 = global read "Meas_global.vi" "Remote control"() -> (w373:bool)
                n201 = Greater?(x=w381, y=1) -> (0:w379:bool[])
                n202 = Or Array Elements(Boolean array=w379) -> (logical OR=w375:bool)
                n203 = Compound Arithmetic op=AND(invert w373, w375, w372) -> (w374:bool)
                n204 = case shown="True" w374 {
                  tunnel: [TRUE FALSE] -> w377
                  frame False {
                  }
                  frame True {
                    n205 = Current VI's Path() -> (path=w387:path)
                    n206 = call "Open_Close_Front_Panel.ph.vi"("Front Panel Window:Open"=TRUE, "VI path"=w387) -> ()  [unwired: 2 out]
                    n207 = One Button Dialog(message="Non Unique symbol names") -> ()  [unwired: 2 out]
                  }
                }
                n208 = Build Array (concatenate)(w378, w377) -> (w376:bool[])
                n209 = And Array Elements(Boolean array=w376) -> (logical AND=w383:bool)
              }
            }
          }
          frame #11 {
            n210 = And(x=w414, y=w413) -> (x .and. y?=w416:bool)
            n211 = case shown="True" w416 {
              tunnel: w418 -> [_ w425]
              tunnel: [FALSE w424] -> w417
              tunnel: [w419 w423] -> w415
              tunnel: w413 -> [w420 _]
              tunnel: w412 -> [_ _]
              frame False {
                n212 = Not(x=w420) -> (.not. x?=w419:bool)
              }
              frame True {
                n213 = for {
                  shift-right: [w444] -> _
                  shift-left: i16[] [] -> [w443]
                  tunnel: w425 -> [w440] mode=indexing
                  tunnel: [w431] -> w426 mode=indexing
                  shift-right: [w439] -> _
                  shift-left: path[] [] -> [w438]
                  n214 = Unbundle By Name(w440) -> ("Ch No"=w441:i16)
                  n215 = Unbundle By Name(w440) -> ("Inst type"=w437:T2, "Calib filename"=w434:path)
                  n216 = Search 1D Array(1D array=w443, element=w441) -> (index of element=w442:i32)  [unwired: 1 out]
                  n217 = Build Array (concatenate)(w443, w441) -> (w444:i16[])
                  n218 = Equal?(x=Inst_type."Fast FID" ("Inst type"), y=w437) -> (x = y?=w430:bool)
                  n219 = case shown="0, Default" w442 {
                    tunnel: w441 -> [w455 _]
                    tunnel: [w451 FALSE ("true")] -> w433
                    frame 0, Default {
                      n220 = Format Into String(format string="The Ch No %d appears more than once", w455) -> (resulting string=w453:string)  [unwired: 2 in, 1 out]
                      n221 = One Button Dialog(message=w453, button name ("OK")="Ok") -> (true=w451:bool)
                    }
                    frame -1 {
                    }
                  }
                  n222 = Search 1D Array(1D array=w438, element=w434) -> (index of element=w435:i32)  [unwired: 1 out]
                  n223 = Greater Or Equal To 0?(x=w435) -> (x >= 0?=w429:bool)
                  n224 = And(x=w430, y=w429) -> (x .and. y?=w428:bool)
                  n225 = case shown="True" w428 {
                    tunnel: [w446 FALSE ("true")] -> w432
                    tunnel: w434 -> [w445 _]
                    frame True {
                      n226 = Format Into String(format string="Calibration file %s is used more than once.", w445) -> (resulting string=w448:string)  [unwired: 2 in, 1 out]
                      n227 = One Button Dialog(message=w448, button name ("OK")="Ok") -> (true=w446:bool)
                    }
                    frame False {
                    }
                  }
                  n228 = Build Array (concatenate)(w438, w434) -> (w439:path[])
                  n229 = Or(x=w433, y=w432) -> (x .or. y?=w431:bool)
                }
                n230 = Or Array Elements(Boolean array=w426) -> (logical OR=w423:bool)
                n231 = Not(x=w423) -> (.not. x?=w424:bool)
              }
            }
          }
          frame #12 {
            n232 = call "Current_Calib_Filenames.vi"("Mode"=App_Global."Read Global") -> ("Calib Filename Out"=w457:path[], "Channel Numbers Out"=w458:i16[])  [unwired: 2 in, 1 out]
            n233 = for {
              tunnel: w461 -> [w472] mode=indexing
              tunnel: w458 -> [w474]
              tunnel: w457 -> [w473]
              tunnel: [w471] -> w460 mode=indexing
              w469 = Inst_type."Cross wire 2"  # Inst type
              n234 = Unbundle By Name(w472) -> ("Inst type"=w464:T2, "Ch No"=w466:i16, "Use Latest"=w467:bool, "Inst type"=w470:T2)
              n235 = Not Equal?(x=w470, y=w469) -> (x != y?=w468:bool)
              n236 = Compound Arithmetic op=AND(w467, w468) -> (w465:bool)
              n237 = Not Equal?(x=Inst_type."Raw voltage" ("Inst type"), y=w464) -> (x != y?=w462:bool)
              n238 = case shown="True" w465 {
                tunnel: w474 -> [_ w485]
                tunnel: w466 -> [_ w484]
                tunnel: w473 -> [_ w482]
                tunnel: w472 -> [w475 w481]
                tunnel: [w475 w480] -> w471
                tunnel: w462 -> [_ w477]
                frame False {
                }
                frame True {
                  n239 = Search 1D Array(1D array=w485, element=w484) -> (index of element=w483:i32)  [unwired: 1 out]
                  n240 = Index Array(array=w482, index=w483) -> (element=w478:path)
                  n241 = Select(t=w478, s=w477, f=path "") -> (s? t:f=w479:path)
                  n242 = Bundle By Name(cluster=w481, "Calib filename"=w479) -> (w480:T13)
                }
              }
            }
          }
          frame #13 {
            n243 = case shown="True" w487 {
              tunnel: w486 -> [w491 w494]
              tunnel: [w491 w493] -> w490
              tunnel: w489 -> [_ _]
              tunnel: w488 -> [_ w492]
              frame False {
              }
              frame True {
                n244 = case shown="\"Run Program\", Default" w492 {
                  tunnel: w494 -> [w496 w504]
                  tunnel: [w495 w504] -> w493
                  frame "Run Program", Default {
                    n245 = for {
                      tunnel: w496 -> [w497] mode=indexing
                      tunnel: [w498] -> w495 mode=indexing
                      n246 = Unbundle By Name(w497) -> ("Calib filename"=w503:path, "Use Latest"=w502:bool, "Ch No"=w501:i16, "Inst type"=w500:T2)
                      n247 = call "Find_calibration_file.vi"("Inst type"=w500, "Ch No"=w501, "Use Latest Calib"=w502, "filename"=w503) -> ("filename out"=w499:path)
                      n248 = Bundle By Name(cluster=w497, "Calib filename"=w499) -> (w498:T13)
                    }
                  }
                  frame "Setup Front Panel" {
                  }
                }
              }
            }
          }
          frame #14 {
            w507 = 0 ("Index")
            n249 = Index Array(array=w509, index=w507) -> (element=w508:T13)
            n250 = Initialize Array(w508, w507) -> (w506:T20)
            n251 = for {
              shift-right: [w517] -> w511
              shift-left: w506 -> [w516]
              shift-right: [w518] -> w512
              shift-left: w506 -> [w520]
              tunnel: w509 -> [w519] mode=indexing
              n252 = Unbundle By Name(w519) -> ("Move channel"=w521:bool)
              n253 = case shown="True" w521 {
                tunnel: w520 -> [w523 w529]
                tunnel: w519 -> [w525 w528]
                tunnel: [w524 w529] -> w518
                tunnel: [w522 w527] -> w517
                tunnel: w516 -> [w522 w526]
                frame False {
                  n254 = Build Array (concatenate)(w523, w525) -> (w524:T20)
                }
                frame True {
                  n255 = Build Array (concatenate)(w526, w528) -> (w527:T20)
                }
              }
            }
            n256 = Build Array (concatenate)(w512, w511) -> (w510:T20)
            n257 = for {
              tunnel: w510 -> [w515] mode=indexing
              tunnel: [w513] -> w505 mode=indexing
              n258 = Bundle By Name(cluster=w515, "Move channel"=FALSE) -> (w513:T13)
            }
          }
          frame #15 {
            n259 = Not Equal?(x=w530, y=w531) -> (x != y?=w532:bool)
            n260 = case shown="True" w532 {
              tunnel: w531 -> [_ w533]
              frame False {
              }
              frame True {
                n261 = local write "Ch & spans choices"(w533) -> ()
              }
            }
          }
          frame #16 {
            n262 = for {
              shift-right: [w543] -> _
              shift-left: string[] [] -> [w544]
              tunnel: [w546] -> w535 mode=indexing
              tunnel: [w540] -> w536 mode=indexing
              tunnel: w537 -> [w542] mode=indexing
              tunnel: [w539] -> w534 mode=indexing
              n263 = Unbundle By Name(w542) -> ("Inst type"=w545:T2)
              n264 = case shown="\"Propeller anemometer\"" w545 {
                tunnel: [w553 w557 w560 w564 w568 w572 w576 "XW" w583 w588 w591 w595] -> w540
                tunnel: ["U" "P" "U" "U" "tau" "U" "U" "W" "U" "C" "T" "T"] -> w547
                tunnel: w544 -> [w554 w558 w562 w566 w570 w574 w578 w580 w585 w589 w593 w597]
                tunnel: [w552 w556 w561 w565 w569 w573 w577 w580 w584 w587 w592 w596] -> w543
                frame "Propeller anemometer" {
                  w553 = "Prop"
                  n265 = Build Array (concatenate)(w554, w553) -> (w552:string[])
                }
                frame "Pressure Transducer" {
                  w557 = "Mano"
                  n266 = Build Array (concatenate)(w558, w557) -> (w556:string[])
                }
                frame "Raw voltage" {
                  w560 = "RV"
                  n267 = Build Array (concatenate)(w562, w560) -> (w561:string[])
                }
                frame "Pitot-static tube" {
                  w564 = "Pitot"
                  n268 = Build Array (concatenate)(w566, w564) -> (w565:string[])
                }
                frame "Preston tube" {
                  w568 = "Preston"
                  n269 = Build Array (concatenate)(w570, w568) -> (w569:string[])
                }
                frame "Hot wire" {
                  w572 = "HW"
                  n270 = Build Array (concatenate)(w574, w572) -> (w573:string[])
                }
                frame "Cross wire 1" {
                  w576 = "XW"
                  n271 = Build Array (concatenate)(w578, w576) -> (w577:string[])
                }
                frame "Cross wire 2" {
                }
                frame "Generic Linear", Default {
                  w583 = "Gen"
                  n272 = Build Array (concatenate)(w585, w583) -> (w584:string[])
                }
                frame "Fast FID" {
                  w588 = "FF"
                  n273 = Build Array (concatenate)(w589, w588) -> (w587:string[])
                }
                frame "Thermocouple" {
                  w591 = "T"
                  n274 = Build Array (concatenate)(w593, w591) -> (w592:string[])
                }
                frame "Cold wire" {
                  w595 = "CW"
                  n275 = Build Array (concatenate)(w597, w595) -> (w596:string[])
                }
              }
              n276 = call "Analyse_string_array.vi"("String array"=w543) -> ("Unique strings"=w551:string[], "Frequency"=w549:i32[])  [unwired: 1 out]
              n277 = Search 1D Array(1D array=w551, element=w540) -> (index of element=w550:i32)  [unwired: 1 out]
              n278 = Index Array(array=w549, index=w550) -> (element=w541:i32)
              n279 = Number To Decimal String(number=w541) -> (decimal integer string=w539:string)  [unwired: 1 out]
              n280 = Concatenate Strings(w539, w540, ":", w547) -> (w546:string)
            }
          }
          frame #17 {
            w606 = T8 {"Colour"=0, "Inst type"=enum."Pitot-static tube", "Inst name"="Manometer voltage", "Symbol"="U", "Code name"="", "Extra Info"="U", "Inst Array"=enum."PWA", "Index"=0, "Voltage Index"=0, "Extra Titles"=[], "Extra Values"=[]}  # Analysis info cluster
            n281 = property on="Ch Name" class="Str"() -> ("Visible"=w607:bool)  [unwired: 2 in, 2 out]
            n282 = for {
              tunnel: [w632] -> w605 mode=indexing
              tunnel: w600 -> [w629] mode=indexing
              tunnel: w603 -> [w621] mode=indexing
              tunnel: T15 {"high limit (10V)"=10.0, "low limit (-10V)"=-10.0, "Ch No"=0, "Var name"="", "Use Latest Calib"=FALSE} ("Ch and Spans") -> [w628]
              tunnel: [w627] -> w599 mode=indexing
              tunnel: w602 -> [w625] mode=indexing
              tunnel: w606 -> [w624]
              tunnel: w601 -> [w618] mode=indexing
              tunnel: w607 -> [w612]
              i -> [w608]
              n283 = Unbundle By Name(w629) -> ("Use Latest"=w622:bool, "high limit (10V)"=w631:sgl, "low limit (-10V)"=w630:sgl, "Ch No"=w623:i16, "Inst type"=w616:T2, "Symbol"=w615:string, "D"=w614:dbl, "Ch Name"=w611:string)
              n284 = Empty String/Path?(string/path=w615) -> (empty?=w619:bool)
              n285 = Select(t=w618, s=w619, f=w615) -> (s? t:f=w617:string)
              n286 = Format Into String(format string="%s (%s)" ("Format String"), w621, w617) -> (resulting string=w610:string)  [unwired: 2 in, 1 out]
              n287 = Select(t=w611, s=w612, f=w610) -> (s? t:f=w609:string)
              n288 = Bundle By Name(cluster=w628, "Use Latest Calib"=w622, "high limit (10V)"=w631, "low limit (-10V)"=w630, "Ch No"=w623, "Var name"=w609) -> (w632:T15)
              n289 = case shown="\"Propeller anemometer\", Default" w616 {
                tunnel: [w635 w638] -> w626
                tunnel: w623 -> [w633 _]
                tunnel: w614 -> [_ w636]
                frame "Propeller anemometer", Default {
                  n290 = Format Into String(format string="Ch %d" ("Format String"), w633) -> (resulting string=w635:string)  [unwired: 2 in, 1 out]
                }
                frame "Preston tube" {
                  n291 = Format Into String(format string="D = %.2f" ("Format String"), w636) -> (resulting string=w638:string)  [unwired: 2 in, 1 out]
                }
              }
              n292 = Bundle By Name(cluster=w624, "Extra Info"=w626, "Inst type"=w616, "Inst name"=w610, "Symbol"=w617, "Code name"=w625, "Inst Array"=Instrument_Array."Analogue", "Index"=w608, "Voltage Index"=w608) -> (w627:T8)
            }
            "Analysis Info cluster" <- w599
            n293 = global write "Meas_global.vi" "Ch & spans"(w605) -> ()
          }
          frame #18 {
            n294 = global read "Meas_global.vi" "Duplicate channels"() -> (w640:i32[])
            n295 = case shown="True" "Select Duplicate Channels" {
              tunnel: w643 -> [_ _]
              tunnel: w641 -> [w651 w674]
              tunnel: w640 -> [w645 w667]
              tunnel: [w644 w666] -> w639
              frame False {
                n296 = for {
                  tunnel: w651 -> [w665] mode=indexing
                  tunnel: [w664] -> w652 mode=indexing
                  n297 = Unbundle By Name(w665) -> ("Inst type"=w664:T2)
                }
                n298 = for {
                  tunnel: w645 -> [w661] mode=indexing
                  tunnel: w652 -> [w663]
                  tunnel: [w662] -> w656 mode=indexing
                  tunnel: [w661] -> w653 mode=indexing
                  n299 = Index Array(array=w663, index=w661) -> (element=w662:T2)
                }
                n300 = Array Size(array=w651) -> (size(s)=w654:i32)
                n301 = Array Max & Min(array=w656) -> (max value=w657:T2, min value=w658:T2)  [unwired: 2 out]
                n302 = Array Max & Min(array=w653) -> (max index (indices)=w655:i32)  [unwired: 3 out]
                n303 = Array Size(array=w645) -> (size(s)=w650:i32)
                n304 = Equal?(x=w657, y=w658) -> (x = y?=w660:bool)
                n305 = Greater?(x=w650, y=1) -> (0:w647:bool)
                n306 = Greater?(x=w654, y=w655) -> (0:w659:bool)
                n307 = Compound Arithmetic op=AND(w647, w660, w659) -> (w646:bool)
                n308 = Select(t=w645, s=w646, f=i32[] [] ("32bit integer")) -> (s? t:f=w644:i32[])
              }
              frame True {
                n309 = for {
                  tunnel: w674 -> [w681] mode=indexing
                  shift-right: [w676] -> w670
                  shift-left: string[] [] -> [w677]
                  tunnel: w667 -> [w679]
                  tunnel: [w675] -> w669 mode=indexing
                  i -> [w680]
                  n310 = Unbundle By Name(w681) -> ("Inst name"=w675:string)
                  n311 = Search 1D Array(1D array=w679, element=w680) -> (index of element=w678:i32)  [unwired: 1 out]
                  n312 = case shown="0, Default" w678 {
                    tunnel: w677 -> [w684 w685]
                    tunnel: w675 -> [w683 _]
                    tunnel: [w682 w685] -> w676
                    frame 0, Default {
                      n313 = Build Array (concatenate)(w684, w683) -> (w682:string[])
                    }
                    frame -1 {
                    }
                  }
                }
                n314 = call "Select_Strings.vi"("Available Ch names"=w669, "Message"="Please select similar instruments whose results columns will be combined", "Selector mode"=T16."Zero or more", "Desired Ch names (in)"=w670) -> ("Ch Indicies Choosen"=w666:i32[])  [unwired: 4 out]
                n315 = local write "Select Duplicate Channels"(FALSE ("Select Local ADAM Channels")) -> ()
              }
            }
            n316 = global write "Meas_global.vi" "Duplicate channels"(w639) -> ()
          }
          frame #19 {
            w690 = u8 0  # Disabled
            n317 = local read "Acquisition Method"() -> (w694:T10)
            n318 = local read "XW Present?"() -> (w692:bool)
            n319 = property on="Cross wire/LDA" class="Enum (strict)"("Visible"=w692) -> ()  [unwired: 2 in, 2 out]
            n320 = case shown="\"Take LDA data\"" "LDA data" {
              tunnel: [w703 w706] -> w696
              tunnel: w697 -> [_ w704]
              tunnel: w698 -> [_ _]
              tunnel: [w703 w705] -> w689
              frame "No LDA data" {
                w702 = FALSE  # Synchronise Analogue channels with LDA
                w703 = u8 2  # Disabled
                n321 = local write "Synchronise Analogue channels with LDA"(w702) -> ()
              }
              frame "Take LDA data" {
                n322 = stacked-sequence {
                  tunnel: [w707 _] -> w706
                  tunnel: [_ w709] -> w705
                  tunnel: w704 -> [_ w710]
                  frame #0 {
                    w707 = u8 0  # Disabled
                  }
                  frame #1 {
                    n323 = Array Size(array=w710) -> (size(s)=w711:i32)
                    n324 = Not Equal To 0?(x=w711) -> (x != 0?=w708:bool)
                    n325 = case shown="False" w708 {
                      tunnel: w708 -> [w713 _]
                      tunnel: [w712 w714] -> w709
                      frame False {
                        w712 = u8 2  # Disabled
                        n326 = local write "Synchronise Analogue channels with LDA"(w713) -> ()
                      }
                      frame True {
                        w714 = u8 0  # Disabled
                      }
                    }
                  }
                }
              }
            }
            n327 = Equal?(x=w694, y=Board_Types."ADC488" ("Board type")) -> (x = y?=w687:bool)
            n328 = case shown="True" w692 {
              tunnel: [w700 "Cross wire"] -> w686
              frame False {
                w700 = T7."2nd component as calculated"  # Cross wire/LDA
              }
              frame True {
              }
            }
            n329 = global write "Meas_global.vi" "Cross wire + or -ve"(w686) -> ()
            n330 = Select(t=w690, s=w687, f=u8 2 ("Disabled")) -> (s? t:f=w688:u8)
            n331 = property on="Trigger mode" class="Enum (strict)"("Disabled"=w688) -> ()  [unwired: 2 in, 2 out]
            n332 = property on="Synchronise Analogue channels with LDA" class="Bool (strict)"("Disabled"=w689) -> ()  [unwired: 2 in, 2 out]
            n333 = property on="LDA set up" class="Clust (strict)"("Disabled"=w696) -> ()  [unwired: 2 in, 2 out]
            n334 = Wait (ms)(milliseconds to wait=u32 100) -> ()  [unwired: 1 out]
          }
          frame #20 {
            n335 = And(x=w720, y=w721) -> (x .and. y?=w719:bool)
            n336 = local read "Synchronise Analogue channels with LDA"() -> (w718:bool)
            n337 = while {
              shift-left: _ -> [w750]
              shift-right: [w751] -> w715
              tunnel: [w752] -> w717
              stop <- FALSE continue-if-true
              n338 = local read "Setup filename selector"() -> (w751:u16)
              n339 = Not Equal?(x=w751, y=w750) -> (x != y?=w752:bool)
            }
            n340 = case shown="True" w718 {
              tunnel: w722 -> [_ w731]
              tunnel: w719 -> [_ w730]
              frame False {
              }
              frame True {
                n341 = local read "Acquisition Method"() -> (w734:T10)
                n342 = local write "Trigger mode"(Trigger_Mode."Trigger Every Block" ("Trigger mode")) -> ()
                n343 = Equal?(x=w734, y=Board_Types."NI-DAQmx" ("Acquisition Method")) -> (x = y?=w733:bool)
                n344 = And(x=w730, y=w733) -> (x .and. y?=w732:bool)
                n345 = case shown="True" w732 {
                  tunnel: w731 -> [_ w739]
                  frame False {
                  }
                  frame True {
                    n346 = for {
                      tunnel: w739 -> [w748] mode=indexing
                      tunnel: [w741] -> w738 mode=indexing
                      n347 = Unbundle By Name(w748) -> ("Inst type"=w747:T2, "Symbol"=w745:string)
                      n348 = Equal?(x=w745, y="Sync") -> (x = y?=w743:bool)
                      n349 = Equal?(x=Inst_type."Raw voltage" ("Inst type"), y=w747) -> (x = y?=w742:bool)
                      n350 = And(x=w742, y=w743) -> (x .and. y?=w741:bool)
                    }
                    n351 = Or Array Elements(Boolean array=w738) -> (logical OR=w737:bool)
                    n352 = case shown="True" w737 {
                      frame False {
                        n353 = One Button Dialog(message="To Perform LDA Sync you must provide a Raw voltage channel having the symbol \"Sync\"") -> ()  [unwired: 2 out]
                      }
                      frame True {
                      }
                    }
                  }
                }
              }
            }
            n354 = case shown="True" w717 {
              tunnel: [FALSE ("exists?") w729] -> w716
              tunnel: w715 -> [_ w727]
              frame False {
              }
              frame True {
                n355 = local read "Setup Paths"() -> (w728:path[])
                n356 = Index Array(array=w728, index=w727) -> (element=w726:path)
                n357 = call "Does_file_exist_(simple).vi"("Pathname"=w726) -> ("exists?"=w729:bool)
              }
            }
            n358 = local write "Read Setup File?"(w716) -> ()
            n359 = Current VI's Path() -> (path=w723:path)
            n360 = call "Close_Panel_and_Abort.vi"("Vi path"=w723, "stop"="stop") -> ()  [unwired: 1 out]
          }
        }
      }
    }
    frame #5 {
      n361 = local read "LDA data"() -> (w758:enum16{"No LDA data", "Take LDA data"})
      n362 = case shown="\"Take LDA data\"" w758 {
        tunnel: [FALSE ("Synchronise Analogue channels with LDA") "Synchronise Analogue channels with LDA"] -> w753
        frame "No LDA data" {
        }
        frame "Take LDA data" {
        }
      }
      n363 = global write "Meas_global.vi" "Synchronise with LDA"(w753) -> ()
      n364 = global write "Meas_global.vi" "LDA data"(w758) -> ()
      n365 = Unbundle By Name("LDA set up") -> ("dimensions"=w756:enum16{"1D", "2D"}, "Arrival spacing"=w755:bool, "Transit time"=w754:bool)
      n366 = global write "Meas_global.vi" "dimensions"(w756) -> ()
      n367 = global write "Meas_global.vi" "Arrival spacing"(w755) -> ()
      n368 = global write "Meas_global.vi" "Transit time"(w754) -> ()
    }
    frame #6 {
      n369 = stacked-sequence {
        seq-local: [_ w790 _ _] -> [_ _ _ w878]
        seq-local: [_ _ w846 _] -> [_ _ _ w877]
        seq-local: [w766 _ _ _] -> [_ _ _ w865]
        tunnel: w763 -> [w765 _ _ w869]
        tunnel: w762 -> [_ _ _ w868]
        tunnel: w761 -> [w764 _ _ _]
        frame #0 {
          n370 = local read "PWA Data"() -> (w767:T1)
          n371 = case shown="\"One Ch PWA\"" w767 {
            tunnel: ["" w776] -> w766
            tunnel: w765 -> [_ w775]
            tunnel: w764 -> [_ w771]
            frame "No PWA Data" {
            }
            frame "One Ch PWA" {
              n372 = Not Equal?(x="Calib_Setup.xls", y=w771) -> (x != y?=w770:bool)
              n373 = case shown="\"Setup Front Panel\"" w775 {
                tunnel: [w780 w783 w786 w789] -> w774
                tunnel: [w779 w782 w785 w788] -> w773
                tunnel: [w778 w781 w784 w787] -> w769
                tunnel: w770 -> [w778 w781 w784 _]
                frame "Show Setup" {
                  w780 = TRUE  # Show Panel?
                  w779 = T4 FALSE  # OK
                }
                frame "Run Program" {
                  w783 = FALSE  # Show Panel?
                  w782 = T4 TRUE  # OK
                }
                frame "Save Current Setup" {
                  w786 = FALSE  # Show Panel?
                  w785 = T4 TRUE  # OK
                }
                frame "Setup Front Panel" {
                  w787 = FALSE  # Check Calib file?
                  w789 = FALSE  # Show Panel?
                  w788 = T4 TRUE  # OK
                }
              }
              n374 = global read "Meas_global.vi" "Pre Setup String"() -> (w777:string)
              n375 = call "PWA_Setup_Panel.vi"("Show Panel?"=w774, "Check Calib file?"=w769, "OK"=w773, "Incoming Setup String"=w777) -> ("Outgoing Setup String"=w776:string)  [unwired: 3 out]
            }
          }
        }
        frame #1 {
          n376 = local read "LDA set up"() -> (w797:T6)
          n377 = global read "Meas_global.vi" "Duplicate channels"() -> (w796:i32[])
          n378 = for {
            N: 3 -> [_]
            tunnel: w797 -> [w813]
            tunnel: "LDA " ("Substring") -> [w810]
            shift-right: [w806] -> w792
            shift-left: "" -> [w807]
            i -> [w814]
            n379 = case shown="2" w814 {
              tunnel: w813 -> [w818 w824 w830]
              tunnel: [w816 w822 w828] -> w812
              tunnel: ["Dimensions" "Arrival spacing" "Transit Time"] -> w811
              frame 0, Default {
                n380 = Unbundle By Name(w818) -> ("dimensions"=w817:enum16{"1D", "2D"})
                n381 = case shown="\"2D\"" w817 {
                  tunnel: ["1D" "2D"] -> w816
                  frame "1D" {
                  }
                  frame "2D" {
                  }
                }
              }
              frame 1 {
                n382 = Unbundle By Name(w824) -> ("Arrival spacing"=w823:bool)
                n383 = case shown="False" w823 {
                  tunnel: ["FALSE" "TRUE"] -> w822
                  frame False {
                  }
                  frame True {
                  }
                }
              }
              frame 2 {
                n384 = Unbundle By Name(w830) -> ("Transit time"=w829:bool)
                n385 = case shown="False" w829 {
                  tunnel: ["FALSE" "TRUE"] -> w828
                  frame False {
                  }
                  frame True {
                  }
                }
              }
            }
            n386 = Concatenate Strings(w810, w811) -> (w809:string)
            n387 = call "Characters_to_string.vi"("Characters to write"=w812, "Label for characters"=w809) -> ("Output string"=w808:string)
            n388 = Concatenate Strings(w807, w808) -> (w806:string)
          }
          n389 = for {
            shift-right: [w801] -> w794
            shift-left: "" -> [w804]
            tunnel: w796 -> [w805] mode=indexing
            n390 = Number To Decimal String(number=w805) -> (decimal integer string=w803:string)  [unwired: 1 out]
            n391 = Concatenate Strings(w804, w803, "; ") -> (w801:string)
          }
          n392 = call "Characters_to_string.vi"("Characters to write"=w794, "Label for characters"="Log_Similar_Measurements_in_the _same_column") -> ("Output string"=w791:string)
          n393 = Concatenate Strings(w792, w791) -> (w790:string)
        }
        frame #2 {
          n394 = global write "Meas_global.vi" "Trigger mode"("Trigger mode") -> ()
          n395 = local read "Cross wire"() -> (w849:T7)
          n396 = global read "Preference_global.vi" "Rig Setup"() -> (w835:string)
          n397 = case shown="\"Free Running\"" "Trigger mode" {
            tunnel: ["Free Running" "Trigger Every Block" "Trigger Every Sample" "Start on Trigger"] -> w844
            frame "Free Running" {
            }
            frame "Trigger Every Block" {
            }
            frame "Trigger Every Sample" {
            }
            frame "Start on Trigger" {
            }
          }
          n398 = Match Pattern(string=w835, regular expression="-") -> (before substring=w834:string)  [unwired: 4 out]
          n399 = property on="PWA Data" class="Enum (strict)"() -> ("Strings []"=w840:string[])  [unwired: 2 in, 2 out]
          n400 = global write "Meas_global.vi" "PWA Data"("PWA Data") -> ()
          n401 = Equal?(x=T7."2nd component multipled by -1" ("Cross wire/LDA"), y=w849) -> (x = y?=w848:bool)
          n402 = case shown="\"EnFlo_Tunnel\"" w834 {
            tunnel: ["" w856] -> w833
            frame "False", Default {
            }
            frame "EnFlo_Tunnel" {
              n403 = call "Characters_to_string.vi"("Characters to write"="FALSE", "Label for characters"="Show_all_EnFlo_Tunnel_Columns") -> ("Output string"=w856:string)
            }
          }
          n404 = Index Array(array=w840, index="PWA Data") -> (element=w839:string)
          n405 = Select(t="TRUE", s=w848, f="FALSE") -> (s? t:f=w851:string)
          n406 = call "Characters_to_string.vi"("Characters to write"=w839, "Label for characters"="Pulsed_Wire_Data" ("Variable name")) -> ("Output string"=w838:string)
          n407 = call "Characters_to_string.vi"("Characters to write"=w851, "Label for characters"="Invert Second Component") -> ("Output string"=w847:string)
          n408 = call "Characters_to_string.vi"("Characters to write"=w844, "Label for characters"="Trigger mode") -> ("Output string"=w842:string)
          n409 = Concatenate Strings(w842, w838, w847, w833) -> (w846:string)
        }
        frame #3 {
          w870 = FALSE  # Show Panel?
          n410 = for {
            tunnel: w868 -> [w883] mode=indexing
            tunnel: [w882] -> w864 mode=indexing
            n411 = Unbundle By Name(w883) -> ("Ch Name"=w882:string)
          }
          n412 = global read "Meas_global.vi" "Pre Setup String"() -> (w871:string)
          n413 = call "Choose_Plug_In_to_Run.vi"("setup"=w869, "Show Panel?"=w870, "Setup String In"=w871) -> ("Setup String Out"=w872:string)  [unwired: 1 out]
          n414 = Array To Spreadsheet String(array=w864, 3:"%s" ("format string")) -> (spreadsheet string=w866:string)  [unwired: 1 out]
          n415 = call "Add_label_to_string.vi"("String to write"=w866, "File Label"="Local ADAM Channels") -> ("Output string"=w879:string)
          n416 = call "Date_and_Time_to_string.vi"() -> ("Date and time (spreadsheet)"=w874:string)
          n417 = global read "Meas_global.vi" "New Setup String"() -> (w873:string)
          n418 = call "Value_to_string.vi"("Value"="Sync Delay Time (ms)", "Label for value"="Sync Delay Time (ms)" ("Label for characters")) -> ("Output string"=w867:string)  [unwired: 1 in]
          n419 = Concatenate Strings(w873, w865, w872, w874, w878, w877, w879, w867) -> (w881:string)
          n420 = global write "Meas_global.vi" "New Setup String"(w881) -> ()
          n421 = global write "LDA_meas_global_1.vi" "Sync Delay Time (ms)"("Sync Delay Time (ms)") -> ()
        }
      }
    }
    frame #7 {
      n422 = local read "Setup File"() -> (w884:path)
      n423 = Strip Path(path=w884) -> (name=→"Setup filename out":string)  [unwired: 1 out]
    }
    frame #8 {
      n424 = case shown="\"Take New Data\"" w887 {
        tunnel: w888 -> [w895 w930]
        tunnel: [w889 w924] -> w886
        frame "Take New Data" {
          n425 = for {
            tunnel: w895 -> [w906] mode=indexing
            shift-right: [w902] -> w892
            shift-left: i16[] [] -> [w904]
            shift-right: [w900] -> w891
            shift-left: path[] [] -> [w901]
            tunnel: [w897] -> w889 mode=indexing
            n426 = Unbundle By Name(w906) -> ("Use Latest"=w899:bool, "Inst type"=w905:T2, "Ch No"=w903:i16, "Calib filename"=w898:path)
            n427 = call "Current_Filepath.vi"("Filename in"=w898, "Data Type"="Calibrations") -> ("Filename Out"=w897:path)
            n428 = case shown="\"Propeller anemometer\", Default" w905 {
              tunnel: w904 -> [w913 w923]
              tunnel: w903 -> [w912 _]
              tunnel: [w911 w923] -> w902
              tunnel: w901 -> [w910 w922]
              tunnel: w898 -> [w909 _]
              tunnel: [w908 w922] -> w900
              tunnel: w899 -> [w907 _]
              frame "Propeller anemometer", Default {
                n429 = case shown="False" w907 {
                  tunnel: w913 -> [w919 w921]
                  tunnel: w912 -> [w918 _]
                  tunnel: [w917 w921] -> w911
                  tunnel: w910 -> [w916 w920]
                  tunnel: w909 -> [w915 _]
                  tunnel: [w914 w920] -> w908
                  frame False {
                    n430 = Build Array (concatenate)(w919, w918) -> (w917:i16[])
                    n431 = Build Array (concatenate)(w916, w915) -> (w914:path[])
                  }
                  frame True {
                  }
                }
              }
              frame "Raw voltage" {
              }
            }
          }
          n432 = call "Current_Calib_Filenames.vi"("Calib Filename"=w891, "Channel Numbers"=w892, "Mode"=App_Global."Write to Global") -> ()  [unwired: 3 out]
        }
        frame "Post Process Raw Data File" {
          n433 = for {
            tunnel: w930 -> [w936] mode=indexing
            tunnel: [w935] -> w924 mode=indexing
            n434 = Unbundle By Name(w936) -> ("Calib filename"=w935:path)
          }
          n435 = global read "Meas_global.vi" "Pre Setup String"() -> (w929:string)
          n436 = call "Get_Characters_from_string.vi"("Input string"=w929, "Variable name"="Skip_Block_Numbers_(eg 1;2;5;12)") -> ("Status"=w927:enum16{"Char in string", "Char not in string"}, "Value"=w926:string)  [unwired: 1 in]
          n437 = case shown="\"Char in string\"" w927 {
            tunnel: w926 -> [w933 _]
            tunnel: [w931 i32[] []] -> w925
            frame "Char in string" {
              n438 = call "Get_array_values_fr_String.vi"("String Value"=w933) -> ("Numeric Array"=w932:dbl[])  [unwired: 1 out]
              n439 = To Long Integer(number=w932) -> (32bit integer=w931:i32[])
            }
            frame "Char not in string" {
            }
          }
          n440 = global write "Meas_global.vi" "Blocks to Skip"(w925) -> ()
        }
      }
      n441 = global write "Meas_global.vi" "Calib files"(w886) -> ()
    }
  }
